vi "DAC Save Results.vi"(8 "error in":errorcluster, 9 "Log Details?":bool, 10 "tdms file":refnum<k34>, 11 "DAC HeatFlow AIV in":refnum<class "DAC HeatFlow Temp.lvclass">) -> (0 "error out":errorcluster)   [LabVIEW 2019, in "DAC.lvlib" / "DAC HeatFlow Temp.lvclass"]
uses:
  DAC HeatFlow Temp.lvclass
  C:/Users/krio/Documents/LV_Projects/test-stand/App/DAC/DAC.lvclass
  DAC.lvclass/DAC.ctl
  DAC HeatFlow Temp.lvclass/DAC HeatFlow Temp.ctl
  DAC.lvclass
  <vilib>/Analysis/NI_AALBase.lvlib
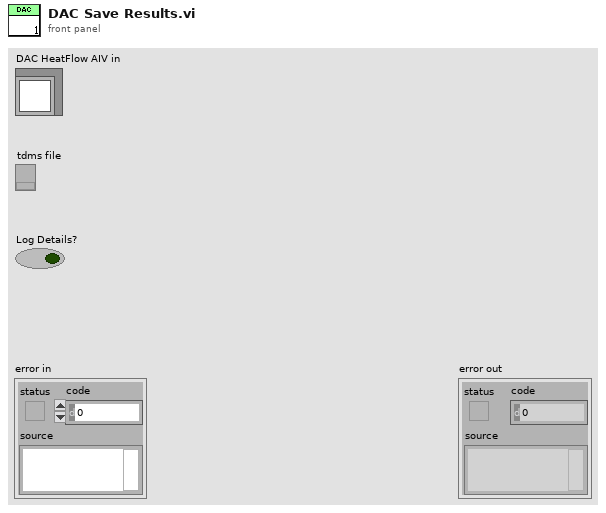
[diagram p1: front panel]
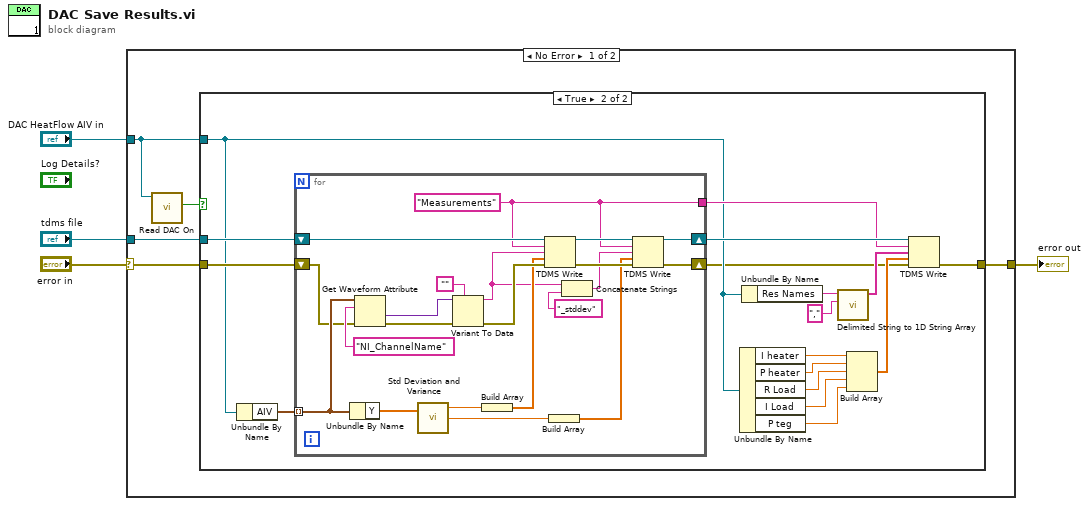
[diagram p0: block diagram]
diagram:
  n1 = case shown="No Error" "error in" {
    selector: "error in" -> [w6 w48]
    tunnel: "DAC HeatFlow AIV in" -> [w9 _]
    tunnel: "tdms file" -> [w7 _]
    tunnel: [w5 w48] -> w1
    frame No Error {
      n2 = call "Read DAC On.vi"("DAC in"=w9) -> ("DAC On"=w8:bool)  [unwired: 8 in, 2 out]
      n3 = case shown="True" w8 {
        tunnel: w9 -> [_ w22]
        tunnel: w7 -> [_ w27]
        tunnel: w6 -> [w10 w25]
        tunnel: [w10 w11] -> w5
        frame False {
        }
        frame True {
          n4 = Unbundle By Name(w22) -> ("AIV"=w26:waveform(dbl)[])
          n5 = for {
            tunnel: w26 -> [w43] mode=indexing
            shift-right: [w39] -> w12
            shift-left: w25 -> [w42]
            shift-right: [w29] -> w24
            shift-left: w27 -> [w47]
            tunnel: [w28] -> w23
            w28 = "Measurements" ("group name in (Untitled)")
            n6 = Unbundle By Name(w43) -> ("Y"=w38:dbl[])
            n7 = Get Waveform Attribute(4:w42, 6:"NI_ChannelName" ("name"), 7:w43) -> (0:w41:errorcluster, 1:w45:variant)  [unwired: 1 in, 2 out]
            n8 = call <vilib>:"Std Deviation and Variance.vi"("X"=w38) -> ("mean"=w37:dbl, "standard deviation"=w35:dbl)  [unwired: 1 in, 1 out]
            n9 = Variant To Data(error in=w41, type="", Variant=w45) -> (data=w32:string, error out=w40:errorcluster)
            n10 = Build Array(w37) -> (w36:dbl[])
            n11 = TDMS Write(0:w47, 5:w28, 7:w32, 9:w36, 11:w40) -> (4:w30:refnum<k34>, 15:w39:errorcluster)  [unwired: 1 in, 2 out]
            n12 = Build Array(w35) -> (w34:dbl[])
            n13 = Concatenate Strings(w32, "_stddev" ("string")) -> (w31:string)
            n14 = TDMS Write(0:w30, 5:w28, 7:w31, 9:w34) -> (4:w29:refnum<k34>)  [unwired: 2 in, 3 out]
          }
          n15 = Unbundle By Name(w22) -> ("I heater"=w18:dbl, "P heater"=w17:dbl, "R Load"=w16:dbl, "I Load"=w15:dbl, "P teg"=w14:dbl)
          n16 = Unbundle By Name(w22) -> ("Res Names"=w20:string)
          n17 = call <vilib>:"Delimited String to 1D String Array.vi"("delimiter"=",", "delimited string"=w20) -> ("string array"=w19:string[])  [unwired: 9 in]
          n18 = Build Array(w18, w17, w16, w15, w14) -> (w13:dbl[])
          n19 = TDMS Write(0:w24, 5:w23, 7:w19, 9:w13, 11:w12) -> (15:w11:errorcluster)  [unwired: 1 in, 3 out]
        }
      }
    }
    frame Error {
    }
  }
  "error out" <- w1
